vi "Save Data.vi"   [LabVIEW 2019]
uses:
  Reusable/Session APIs/File Access/Config Data/Config Session.ctl
  Reusable/Session APIs/File Access/Config Data/Config Data.lvclass
  C:/Program Files (x86)/National Instruments/LabVIEW 2019/vi.lib/MSR Consulting, LLC/General Reuse/Session APIs/_Session Fwk/Session - Root.lvclass
  Reusable/Session APIs/File Access/Config Data/Config Data.lvclass/Config Data.ctl
  CRD/Data/Open Path Data.lvclass
  Z:/sw_repo/handix/source/Reusable/Data/Data.lvclass
  Z:/sw_repo/handix/source/Reusable/CRDS/Data/Main/CRDS Data.lvclass
  Devices/Alicat/Session Based/Data/Alicat Data.lvclass
  Devices/CR5/Data/CR5 Data.lvclass
  Reusable/CRDS/Data/Cell/CRDS Cell Data.lvclass
  CRD/Data/Open Path Data.lvclass/Open Path Data.ctl
  Reusable/CRDS/Data/Cell/CRDS Cell Data.lvclass/CRDS Cell Data.ctl
  Devices/CR5/Data/CR5 Data.lvclass/CR5 Data.ctl
  CRD/Data/Read Alicat Data.vi
  CRD/Data/Accessors/Read CR5.vi
  CRD/Data/Accessors/Read Heated Line Temp.vi
  CRD/Data/Accessors/Read Thermistor Data.vi
  CRD/Data/Accessors/Read u.vi
  CRD/Data/Accessors/Read VaisalaDuct.vi
  CRD/Data/Accessors/Read VaisalaOutside.vi
  CRD/Data/Accessors/Read Pressure.vi
  Devices/CR5/Data/Accessors/Read Balance.vi
  Devices/CR5/Data/Accessors/Read flag.vi
  Devices/CR5/Data/Accessors/Read mirror flag.vi
  Devices/CR5/Data/Accessors/Read PWM.vi
  Devices/CR5/Data/Accessors/Read Tamb.vi
  Devices/CR5/Data/Accessors/Read Tboard.vi
  Devices/CR5/Data/Accessors/Read Tmirror.vi
  Reusable/CRDS/Data/Cell/Read extParam.vi
  Reusable/Session APIs/File Access/Config Data/Accessors/Write Cfg Path.vi
  Reusable/Session APIs/File Access/Config Data/Accessors/Read Ref.vi
  <vilib>/Utility/config.llb/Read Key (Boolean).vi
  <vilib>/Utility/config.llb/Read Key (I32).vi
  <vilib>/Utility/config.llb/Read Key (String).vi
  <vilib>/Utility/config.llb/Read Key (Path).vi
  Reusable/Data/Read measTime.vi
  Reusable/CRDS/Data/Main/Read CellData.vi
  Reusable/CRDS/Data/Main/Read filter.vi
  Reusable/File IO/File Utilities.lvlib
  <vilib>/nisyscfg/nisyscfg.lvlib
  <vilib>/MSR Consulting, LLC/General Reuse/Session APIs/_Session Fwk/Session - Root.lvclass
  <vilib>/Utility/config.llb/NI_LVConfig.lvlib
types:
  T1 = typedef "Config Data.lvclass/Config Session.ctl" = refnum<data-value>
  T2 = typedef "Session - Root.lvclass/Session Handle.ctl" = refnum<data-value>
  T3 = typedef "NI_LVConfig.lvlib/Config Data RefNum.ctl" = refnum<k1>
  T4 = typedef "extparam.ctl" = cluster{"Tau":sgl, "Tau0cor":sgl, "ext":sgl, "extCorr":sgl, "stdevTau":sgl, "eTau":sgl, "taucorr":sgl, "Tau0":sgl, "max":sgl}
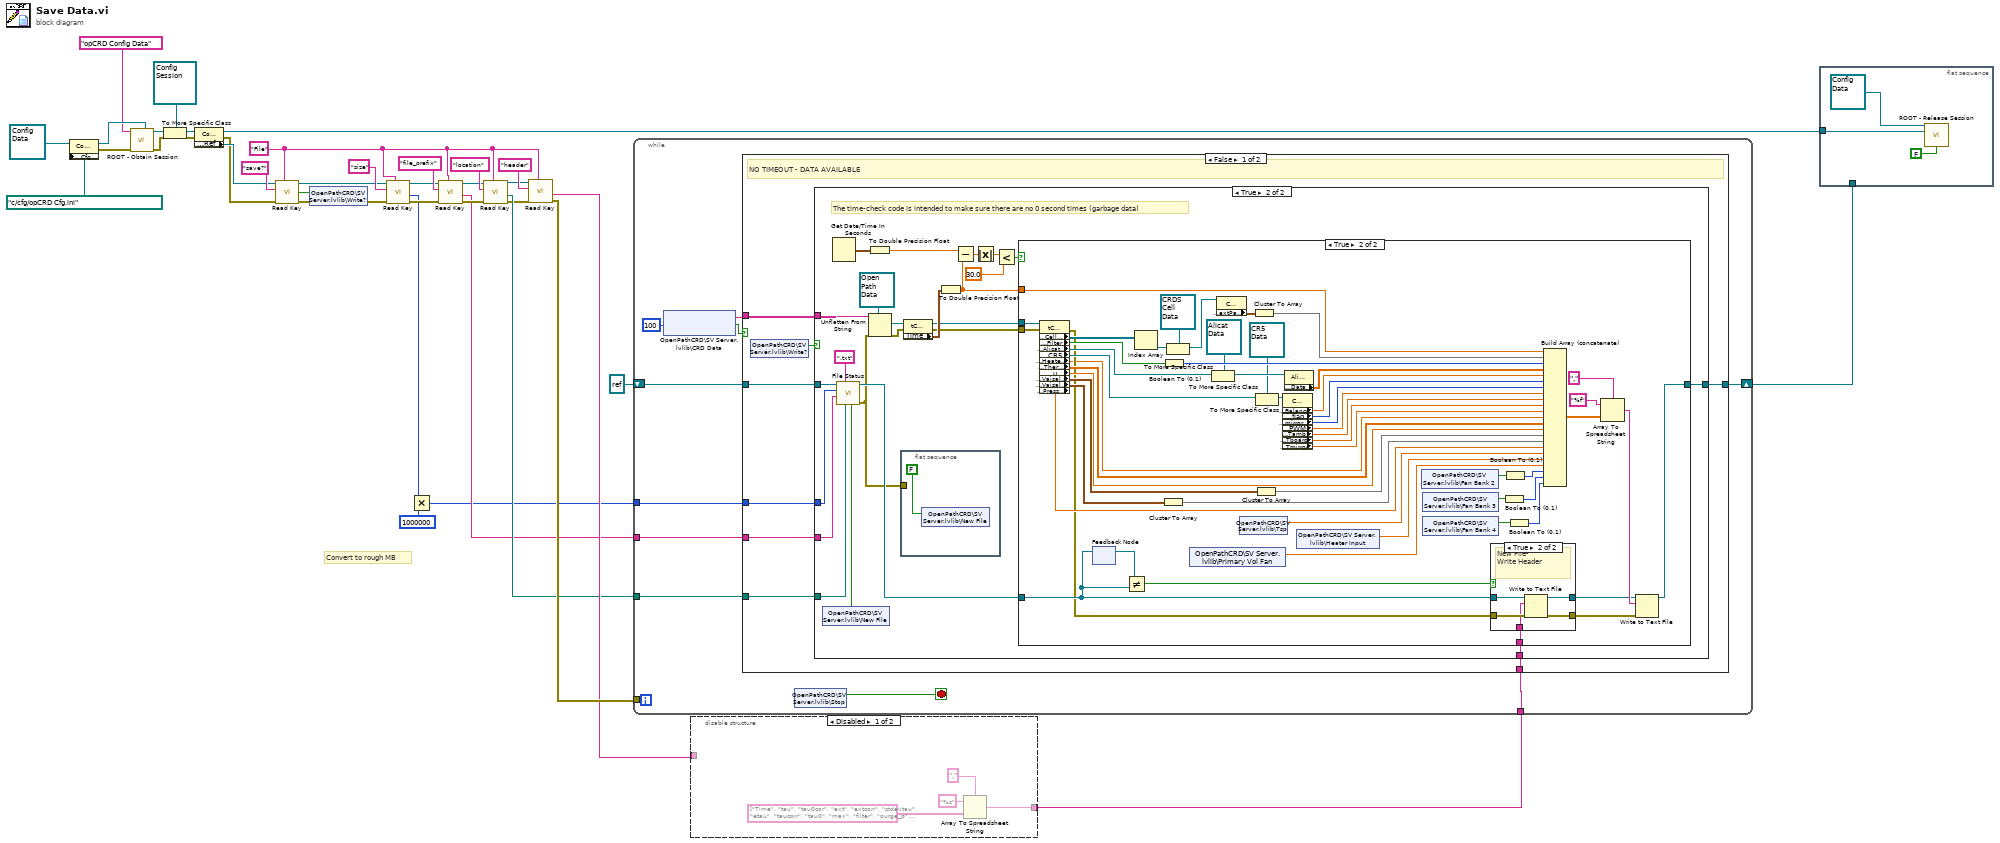
[diagram p0: block diagram]
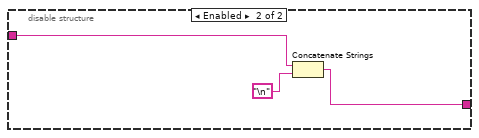
[diagram p2: hidden frame]
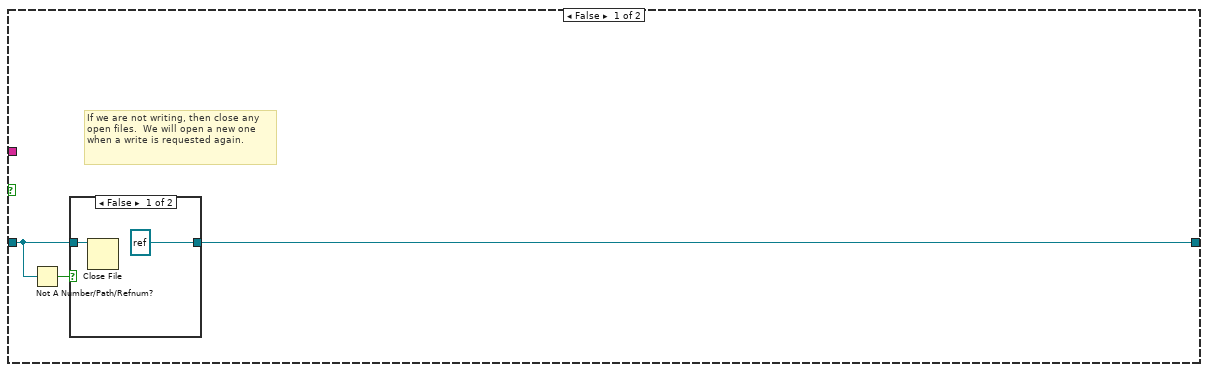
[diagram p3: hidden frame]
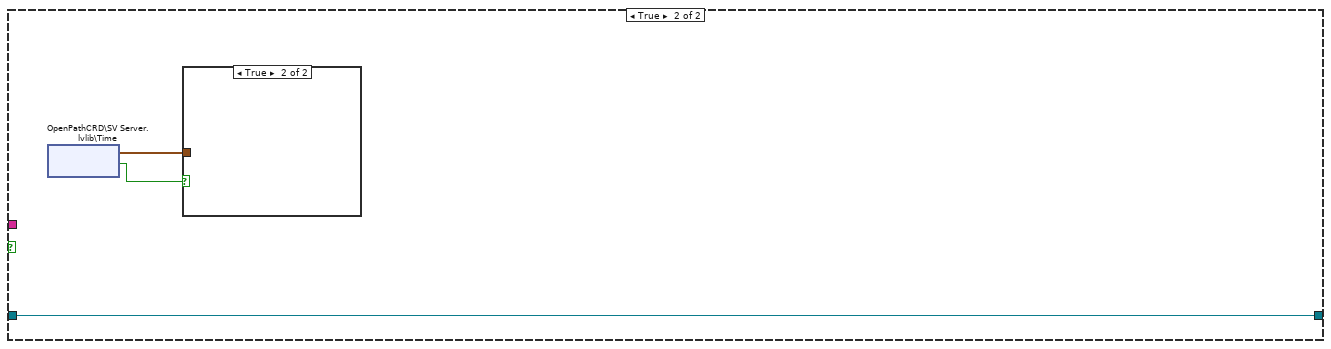
[diagram p7: hidden frame]
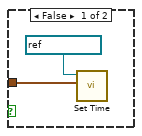
[diagram p8: hidden frame]
diagram:
  w3 = "File" ("section")
  # "Convert to rough MB"
  n1 = property class="Config Data"(reference=refnum<class "Config Data.lvclass"> refnum ("Config Data"), "Accessors:Cfg Path"=path "c:/cfg/opCRD Cfg.ini" ("Path")) -> (reference out=w16:refnum<class "Config Data.lvclass">, error out=w15:errorcluster)  [unwired: 1 in]
  n2 = call <vilib>:"ROOT - Obtain Session.vi"("Session Name ()"="opCRD Config Data", "OBJ - Session"=w16, "error in (no error)"=w15) -> ("Session Handle"=w17:T2, "error out"=w18:errorcluster)  [unwired: 10 in, 1 out]
  n3 = To More Specific Class(target class=T1 refnum ("Session Handle"), reference=w17, error in=w18) -> (specific class reference=w8:T1, error out=w39:errorcluster)
  n4 = property class="Config Data"(reference=w8, error in=w39) -> (reference out=w7:T1, error out=w6:errorcluster, "Accessors:Ref"=w19:T3)
  n5 = call-poly <vilib>:"Read Key.vi"("section"=w3, "error in (no error)"=w6, "key"="save?", "refnum"=w19) -> ("error out"=w5:errorcluster, "value"=w21:bool, "refnum out"=w22:T3)  [unwired: 4 in, 1 out]
  n6 = shared-variable "OpenPathCRD\\SV Server.lvlib\\Write?"(w21, error in=w5) -> (error out=w4:errorcluster)
  n7 = call-poly <vilib>:"Read Key.vi"("section"=w3, "error in (no error)"=w4, "key"="size", "refnum"=w22) -> ("error out"=w33:errorcluster, "value"=w24:i32, "refnum out"=w27:T3)  [unwired: 4 in, 1 out]
  n8 = Multiply(x=w24, y=1000000) -> (x*y=w26:i32)
  n9 = call-poly <vilib>:"Read Key.vi"("section"=w3, "error in (no error)"=w33, "key"="file_prefix", "refnum"=w27) -> ("error out"=w34:errorcluster, "value"=w29:string, "refnum out"=w30:T3)  [unwired: 4 in, 1 out]
  n10 = call-poly <vilib>:"Read Key.vi"("section"=w3, "error in (no error)"=w34, "key"="location", "refnum"=w30) -> ("error out"=w2:errorcluster, "value"=w32:path, "refnum out"=w35:T3)  [unwired: 4 in, 1 out]
  n11 = call-poly <vilib>:"Read Key.vi"("section"=w3, "error in (no error)"=w2, "key"="header", "refnum"=w35) -> ("error out"=w38:errorcluster, "value"=w37:string)  [unwired: 4 in, 2 out]
  n12 = disable-structure shown="Disabled" {
    disable-tunnel: [w40 w44] -> w10
    disable-tunnel: w37 -> [_ w46]
    frame Disabled {
      n13 = Array To Spreadsheet String(delimiter (Tab)=",", array=string[] ["Time", "tau", "tau0cor", "ext", "extcorr", "stdevtau", "etau", "taucorr", "tau0", "max", "filter", "purge_p", "purge_T", "purge_Q", "purge_Q0", "purge_Qsp", "cr5_balance", "cr5_flag", "cr5_mirror_flag", "cr5_pwm", "cr5_Tamb", "cr5_Tboard", "cr5_Tmirror", "Theatedline", "Thermistor_1", "Thermistor_2", "u", "vaisala_RH_duct", "vaisala_T_duct", "vaisala_RH_ambient", "vaisala_T_ambient", "Pressure", "T_heated_SP"], 3:"%s" ("format string")) -> (spreadsheet string=w40:string)
    }
    frame Enabled {
      n14 = Concatenate Strings(w46, "\n") -> (w44:string)
    }
  }
  n15 = while {
    shift-right: [w51] -> w1
    shift-left: refnum<file> refnum ("fileRefIn") -> [w52]
    tunnel: w10 -> [w50]
    tunnel: w26 -> [w49]
    tunnel: w29 -> [w48]
    tunnel: w32 -> [w47]
    tunnel: w38 -> [_]
    stop <- w56 stop-if-true
    n16 = shared-variable "OpenPathCRD\\SV Server.lvlib\\CRD Data"(100 ("ms timeout (0)")) -> (w53:string, w54:bool)  [unwired: 1 in, 1 out]
    n17 = case shown="False" w54 {
      tunnel: w53 -> [w64 _]
      tunnel: w52 -> [w63 w160]
      tunnel: [w62 w160] -> w51
      tunnel: w50 -> [w60 _]
      tunnel: w49 -> [w59 _]
      tunnel: w48 -> [w58 _]
      tunnel: w47 -> [w57 _]
      frame False {
        # "NO TIMEOUT - DATA AVAILABLE"
        n18 = shared-variable "OpenPathCRD\\SV Server.lvlib\\Write?"() -> (w61:bool)  [unwired: 1 in, 1 out]
        n19 = case shown="True" w61 {
          tunnel: w64 -> [_ w94]
          tunnel: w63 -> [w66 w91]
          tunnel: [w65 w90] -> w62
          tunnel: w60 -> [_ w89]
          tunnel: w59 -> [_ w88]
          tunnel: w58 -> [_ w87]
          tunnel: w57 -> [_ w86]
          frame False {
            # "If we are not writing, then close any open files.  We will open a new one when a write is requested again."
            n20 = Not A Number/Path/Refnum?(number/path/refnum=w66) -> (NaN/Path/Refnum?=w67:bool)
            n21 = case shown="False" w67 {
              tunnel: w66 -> [w69 w70]
              tunnel: [refnum<file> refnum ("refnum out") w70] -> w65
              frame False {
                n22 = Close File(refnum=w69) -> ()  [unwired: 1 in, 2 out]
              }
              frame True {
              }
            }
          }
          frame True {
            # "The time-check code is intended to make sure there are no 0 second times (garbage data)"
            n23 = shared-variable "OpenPathCRD\\SV Server.lvlib\\New File"() -> (w72:bool)  [unwired: 1 in, 1 out]
            n24 = Get Date/Time In Seconds() -> (seconds since 1Jan1904=w75:timestamp)
            n25 = call "File Status.vi"("nFile"=w72, "Data Path"=w86, "ext"=".txt", "prefix"=w87, "fSize"=w88, "fileRefIn"=w91) -> ("error out"=w71:errorcluster, "fileRefOut"=w80:refnum<file>)  [unwired: 3 in, 1 out]
            n26 = To Double Precision Float(number=w75) -> (double precision float=w74:dbl)
            n27 = Unflatten From String(type=refnum<class "Open Path Data.lvclass"> refnum ("tCRD Data"), binary string=w94, error in (no error)=w71) -> (value=w78:refnum<class "Open Path Data.lvclass">, error out=w79:errorcluster)  [unwired: 2 in, 1 out]
            n28 = flat-sequence {
              tunnel: w71 -> [_]
              frame #0 {
                n29 = shared-variable "OpenPathCRD\\SV Server.lvlib\\New File"(FALSE) -> ()  [unwired: 1 in, 1 out]
              }
            }
            n30 = property class="tCRD Data"(reference=w78, error in=w79) -> (reference out=w77:refnum<class "Open Path Data.lvclass">, error out=w73:errorcluster, "Time"=w85:timestamp)
            n31 = To Double Precision Float(number=w85) -> (double precision float=w76:dbl)
            n32 = Subtract(x=w74, y=w76) -> (x-y=w84:dbl)
            n33 = Absolute Value(x=w84) -> (abs(x)=w83:dbl)
            n34 = Less?(x=w83, y=30.0) -> (x < y?=w81:bool)
            n35 = case shown="True" w81 {
              tunnel: w76 -> [_ w146]
              tunnel: [w96 w143] -> w90
              tunnel: w89 -> [_ w138]
              tunnel: w80 -> [w96 w112]
              tunnel: w77 -> [_ w110]
              tunnel: w73 -> [_ w100]
              frame False {
              }
              frame True {
                n36 = property class="tCRD Data"(reference=w110, error in=w100) -> (error out=w99:errorcluster, "Data Access:Cell Data"=w109:refnum<class "CRDS Cell Data.lvclass">[], "Data Access:Filter"=w108:bool, "Accessors:Alicat Data"=w107:refnum<class "Alicat Data.lvclass">, "Accessors:CR5"=w106:refnum<class "CR5 Data.lvclass">, "Accessors:Heated Line Temp"=w98:dbl, "Accessors:Thermistor Data"=w105:dbl[], "Accessors:u"=w104:sgl, "Accessors:VaisalaDuct"=w103:cluster{"RH":sgl, "T":sgl}, "Accessors:VaisalaOutside"=w102:cluster{"RH":sgl, "T":sgl}, "Accessors:Pressure"=w101:dbl)  [unwired: 1 out]
                n37 = feedback-in #1(w112) -> ()
                n38 = feedback #1() -> (w114:refnum<file>)  [unwired: 1 in]
                n39 = Not Equal?(x=w114, y=w112) -> (x != y?=w113:bool)
                n40 = Index Array(array=w109) -> (element=w150:refnum<class "CRDS Cell Data.lvclass">)  [unwired: 1 in]
                n41 = Cluster To Array(cluster=w102) -> (array=w124:sgl[])
                n42 = Boolean To (0,1)(Boolean=w108) -> (0, 1=w145:i16)
                n43 = To More Specific Class(target class=refnum<class "CRDS Cell Data.lvclass"> refnum ("CRDS Cell"), reference=w150) -> (specific class reference=w149:refnum<class "CRDS Cell Data.lvclass">)  [unwired: 1 in, 1 out]
                n44 = shared-variable "OpenPathCRD\\SV Server.lvlib\\Primary Vol Fan"() -> (w121:dbl)  [unwired: 1 in, 1 out]
                n45 = To More Specific Class(target class=refnum<class "Alicat Data.lvclass"> refnum ("Alicat Data"), reference=w107) -> (specific class reference=w136:refnum<class "Alicat Data.lvclass">)  [unwired: 1 in, 1 out]
                n46 = property class="CRDS Cell"(reference=w149) -> ("Data Access:extParam"=w148:T4)  [unwired: 1 in, 2 out]
                n47 = shared-variable "OpenPathCRD\\SV Server.lvlib\\Tsp"() -> (w111:dbl)  [unwired: 1 in, 1 out]
                n48 = Cluster To Array(cluster=w148) -> (array=w147:sgl[])
                n49 = Cluster To Array(cluster=w103) -> (array=w125:sgl[])
                n50 = To More Specific Class(target class=refnum<class "CR5 Data.lvclass"> refnum ("CR5 Data"), reference=w106) -> (specific class reference=w133:refnum<class "CR5 Data.lvclass">)  [unwired: 1 in, 1 out]
                n51 = property class="CR5 Data"(reference=w133) -> ("Accessors:Balance"=w132:dbl, "Accessors:flag"=w131:i32, "Accessors:mirror flag"=w130:i32, "Accessors:PWM"=w129:dbl, "Accessors:Tamb"=w128:dbl, "Accessors:Tboard"=w127:dbl, "Accessors:Tmirror"=w126:dbl)  [unwired: 1 in, 2 out]
                n52 = property class="Alicat Data"(reference=w136) -> ("Accessors:Data"=w135:sgl[])  [unwired: 1 in, 2 out]
                n53 = shared-variable "OpenPathCRD\\SV Server.lvlib\\Heater Input"() -> (w122:dbl)  [unwired: 1 in, 1 out]
                n54 = shared-variable "OpenPathCRD\\SV Server.lvlib\\Fan Bank 2"() -> (w120:bool)  [unwired: 1 in, 1 out]
                n55 = shared-variable "OpenPathCRD\\SV Server.lvlib\\Fan Bank 3"() -> (w118:bool)  [unwired: 1 in, 1 out]
                n56 = shared-variable "OpenPathCRD\\SV Server.lvlib\\Fan Bank 4"() -> (w116:bool)  [unwired: 1 in, 1 out]
                n57 = case shown="True" w113 {
                  tunnel: w112 -> [w152 w157]
                  tunnel: [w152 w156] -> w97
                  tunnel: w99 -> [w151 w155]
                  tunnel: [w151 w154] -> w144
                  tunnel: w138 -> [_ w153]
                  frame False {
                  }
                  frame True {
                    # "New File-\nWrite Header"
                    n58 = Write to Text File(file (use dialog)=w157, text=w153, error in=w155) -> (refnum out=w156:refnum<file>, error out=w154:errorcluster)  [unwired: 1 in, 1 out]
                  }
                }
                n59 = Boolean To (0,1)(Boolean=w118) -> (0, 1=w117:i16)
                n60 = Boolean To (0,1)(Boolean=w120) -> (0, 1=w119:i16)
                n61 = Boolean To (0,1)(Boolean=w116) -> (0, 1=w115:i16)
                n62 = Build Array (concatenate)(w146, w147, w145, w135, w132, w131, w130, w129, w128, w127, w126, w98, w105, w104, w125, w124, w101, w111, w122, w121, w119, w117, w115) -> (w142:dbl[])
                n63 = Array To Spreadsheet String(delimiter (Tab)=",", array=w142, 3:"%f" ("format string")) -> (spreadsheet string=w139:string)
                n64 = Write to Text File(file (use dialog)=w97, text=w139, error in=w144) -> (refnum out=w143:refnum<file>)  [unwired: 1 in, 2 out]
              }
            }
          }
        }
      }
      frame True {
        n65 = shared-variable "OpenPathCRD\\SV Server.lvlib\\Time"() -> (w159:timestamp, w158:bool)  [unwired: 2 in, 1 out]
        n66 = case shown="True" w158 {
          tunnel: w159 -> [w162 _]
          frame False {
            n67 = call <vilib>:"Set Time.vi"("Time"=w162, "Session in (localhost)"=refnum<k21> "localhost") -> ()  [unwired: 6 in, 4 out]
          }
          frame True {
          }
        }
      }
    }
    n68 = shared-variable "OpenPathCRD\\SV Server.lvlib\\Stop"() -> (w56:bool)  [unwired: 1 in, 1 out]
  }
  n69 = flat-sequence {
    tunnel: w7 -> [w163]
    tunnel: w1 -> [_]
    frame #0 {
      n70 = call <vilib>:"ROOT - Release Session.vi"("OBJ - Session in"=refnum<class "Config Data.lvclass"> refnum ("Config Data"), "Session Handle in"=w163, "force destroy? (F)"=FALSE) -> ()  [unwired: 11 in, 2 out]
    }
  }
